vi "find chanelsenser.vi"(11 "configtable":T1 {"CHS"."display" format="%b"}) -> (3 "senser out":string[](array[string]))   [LabVIEW 2011]
uses:
  contable.ctl
  CHS.ctl
  singlechtype.ctl
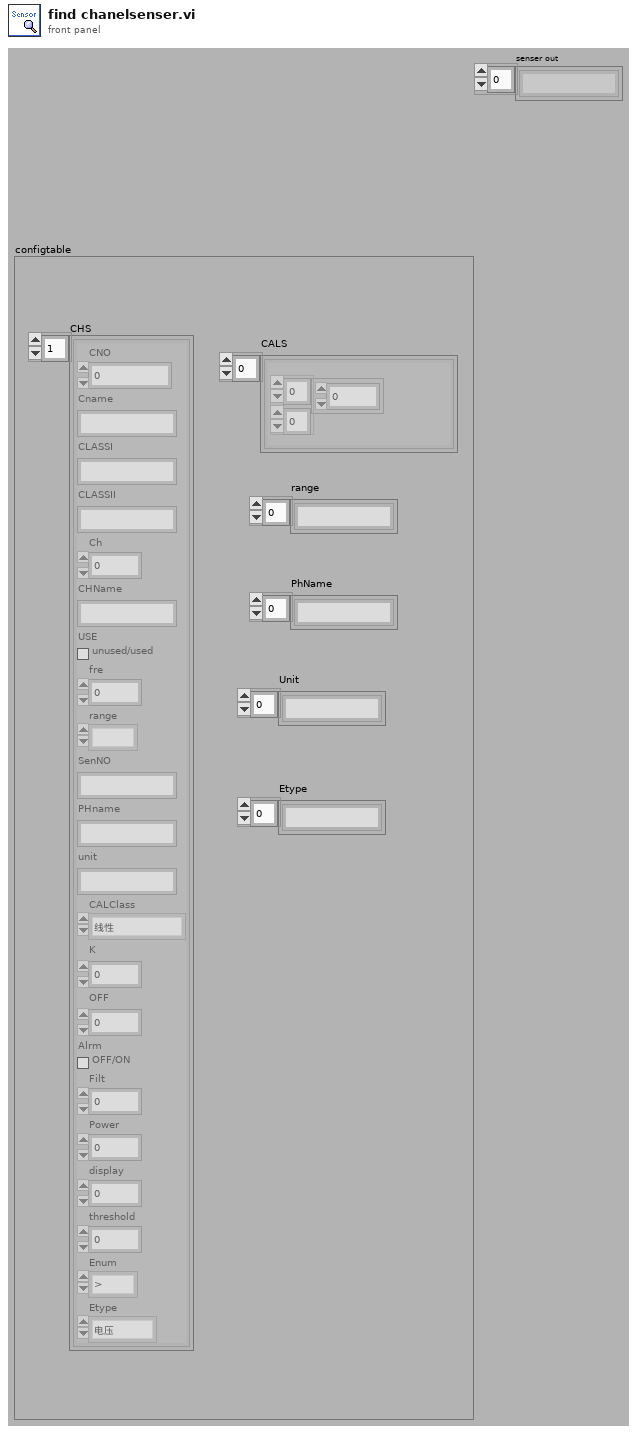
[diagram p1: front panel]
types:
  T1 = typedef "contable.ctl" = cluster{"CHS":T2, "CALS":cluster{"Array":dbl[][]}[], "range":string[], "PhName":string[], "Unit":string[], "Etype":string[]}
  T2 = typedef "CHS.ctl" = T3[]
  T3 = typedef "singlechtype.ctl" = cluster{"CNO":u8, "Cname":string, "CLASSI":string, "CLASSII":string, "Ch":u8, "CHName":string, "USE":bool, "fre":dbl, "range":enum16{""}, "SenNO":string, "PHname":string, "unit":string, "CALClass":enum8{"线性", "查表", "公式"}, "K":dbl, "OFF":dbl, "Alrm":bool, "Filt":dbl, "Power":u8, "display":u8, "threshold ":dbl, "Enum":enum16{">", ">=", "<", "<=", "<>(在范围内）", "><（在范围外）"}, "Etype":enum16{"电压", "电流", "电阻", "热电偶K", "热电偶T"}}
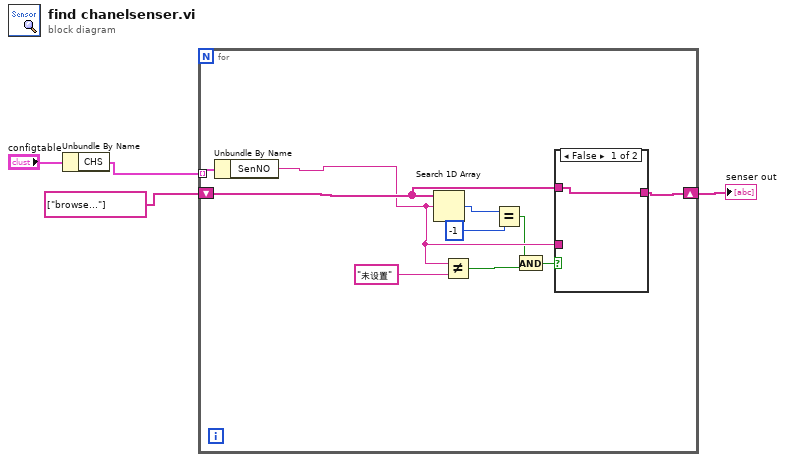
[diagram p0: block diagram]
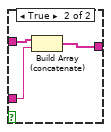
[diagram p2: hidden frame]
diagram:
  n1 = Unbundle By Name("configtable") -> ("CHS"=w1:T2)
  n2 = for {
    tunnel: w1 -> [w14] mode=indexing
    shift-right: [w12] -> w2
    shift-left: string[] ["browse..."] -> [w13]
    n3 = Unbundle By Name(w14) -> ("SenNO"=w11:string)
    n4 = Search 1D Array(1D array=w13, element=w11) -> (index of element=w10:i32)  [unwired: 1 out]
    n5 = Not Equal?(x=w11, y="未设置") -> (x != y?=w6:bool)
    n6 = Equal?(x=w10, y=-1) -> (x = y?=w7:bool)
    n7 = And(x=w7, y=w6) -> (x .and. y?=w5:bool)
    n8 = case shown="False" w5 {
      tunnel: w13 -> [w15 w18]
      tunnel: [w15 w17] -> w12
      tunnel: w11 -> [_ w16]
      frame False {
      }
      frame True {
        n9 = Build Array (concatenate)(w18, w16) -> (w17:string[])
      }
    }
  }
  "senser out" <- w2
